vi "Initialise Panel.vi"(8 "error in":errorcluster, 9 "MHL Configuration":T6, 10 "MHL References":T5, 11 "MHL UI Data In":T2={"Status"="", "Connection Type"=enum."Ethernet", "Connected to Controller"=FALSE, "Axes Enabled"=FALSE, "Jogging Enabled"=FALSE, "X Axis MPOS"=0.0, "A Axis MPOS"=0.0, "X Axis SPEED"=0.0, "A Axis SPEED"=0.0, "Plot Laser Data"=FALSE, "MHL Status"=enum."Disconnected"} {"A Axis SPEED" format="%#_4g"; "X Axis SPEED" format="%#_4g"; "A Axis MPOS" format="%#_4g"; "X Axis MPOS" format="%#_4g"}) -> (0 "error out":errorcluster, 2 "MHL Data":T1={"MHL UI Data"={"Status"="", "Connection Type"=enum."Ethernet", "Connected to Controller"=FALSE, "Axes Enabled"=FALSE, "Jogging Enabled"=FALSE, "X Axis MPOS"=0.0, "A Axis MPOS"=0.0, "X Axis SPEED"=0.0, "A Axis SPEED"=0.0, "Plot Laser Data"=FALSE, "MHL Status"=enum."Disconnected"}, "MHL References"={"Connect to Controller Ref"=refnum, "Connection Type Ref"=refnum, "Set Parameters Ref"=refnum, "Enable Axes Ref"=refnum, "Home Axes Ref"=refnum}, "MHL Configuration"={"Fuel Control Valve Maximum"=0.0, "Fuel Control Valve Minimum"=0.0}} {"MHL UI Data"."A Axis SPEED" format="%#_4g"; "MHL UI Data"."X Axis SPEED" format="%#_4g"; "MHL UI Data"."A Axis MPOS" format="%#_4g"; "MHL UI Data"."X Axis MPOS" format="%#_4g"}, 3 "MHL UI Data Out":T2={"Status"="", "Connection Type"=enum."Ethernet", "Connected to Controller"=FALSE, "Axes Enabled"=FALSE, "Jogging Enabled"=FALSE, "X Axis MPOS"=0.0, "A Axis MPOS"=0.0, "X Axis SPEED"=0.0, "A Axis SPEED"=0.0, "Plot Laser Data"=FALSE, "MHL Status"=enum."Disconnected"} {"A Axis SPEED" format="%#_4g"; "X Axis SPEED" format="%#_4g"; "A Axis MPOS" format="%#_4g"; "X Axis MPOS" format="%#_4g"})   [LabVIEW 2020]
uses:
  controls/MHL UI Data.ctl
  TrioMotion Controller/Connection Type.ctl
  controls/MHL Status.ctl
  controls/MHL Configuration.ctl
  controls/MHL References.ctl
  controls/MHL Data.ctl
  SR-Test Med System Globals.vi
  TrioMotion Controller/TrioMotion Controller.lvlib
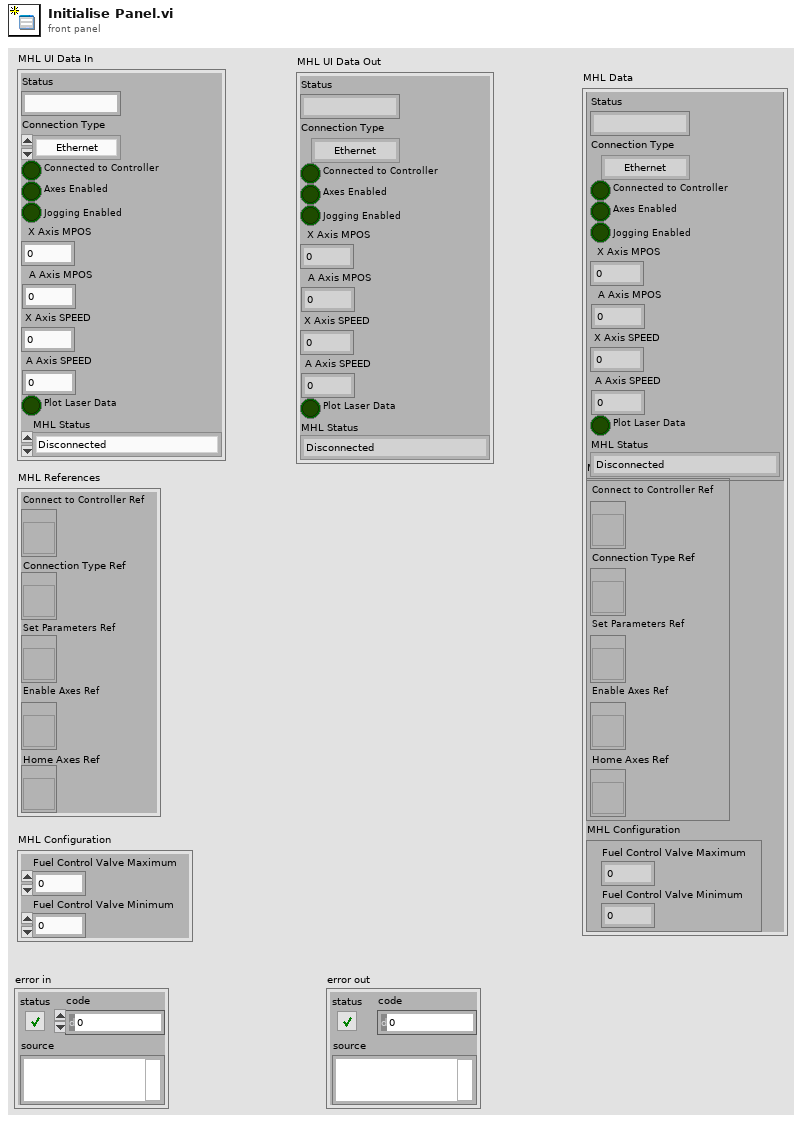
[diagram p1: front panel]
types:
  T1 = typedef "MHL Data.ctl" = cluster{"MHL UI Data":T2, "MHL References":T5, "MHL Configuration":T6}
  T2 = typedef "MHL UI Data.ctl" = cluster{"Status":string, "Connection Type":T3, "Connected to Controller":bool, "Axes Enabled":bool, "Jogging Enabled":bool, "X Axis MPOS":dbl, "A Axis MPOS":dbl, "X Axis SPEED":dbl, "A Axis SPEED":dbl, "Plot Laser Data":bool, "MHL Status":T4}
  T3 = typedef "TrioMotion Controller.lvlib/Connection Type.ctl" = enum16{"USB", "Serial", "Ethernet", "PCI", "Path", "No connection"}
  T4 = typedef "MHL Status.ctl" = enum16{"Disconnected", "Connecting", "Connected", "Axes Enabled", "Machine Running", "Shutdown"}
  T5 = typedef "MHL References.ctl" = cluster{"Connect to Controller Ref":refnum<vi>, "Connection Type Ref":refnum<vi>, "Set Parameters Ref":refnum<vi>, "Enable Axes Ref":refnum<vi>, "Home Axes Ref":refnum<vi>}
  T6 = typedef "MHL Configuration.ctl" = cluster{"Fuel Control Valve Maximum":dbl, "Fuel Control Valve Minimum":dbl}
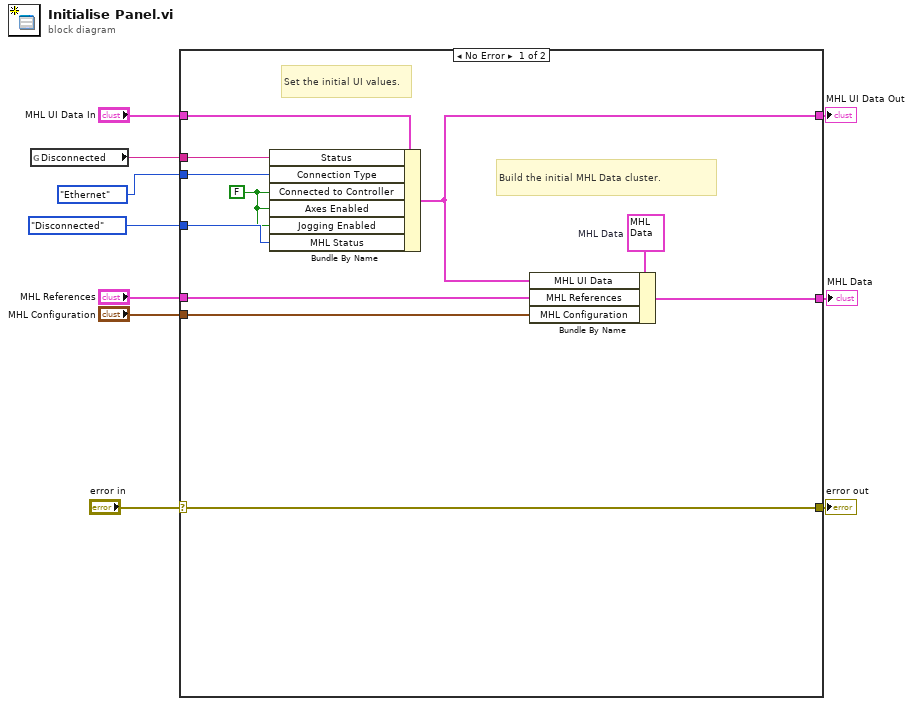
[diagram p0: block diagram]
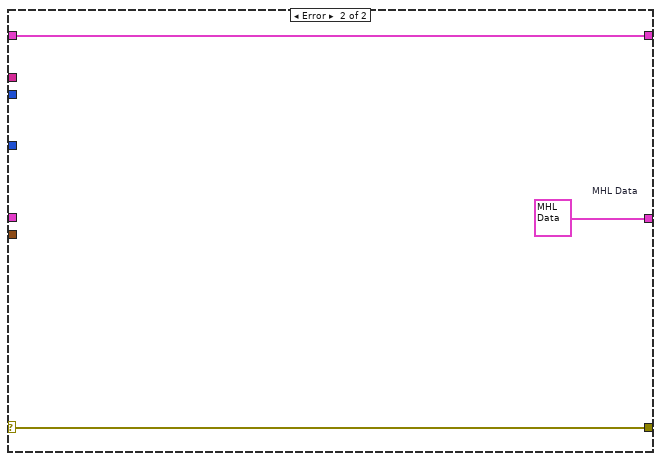
[diagram p2: hidden frame]
diagram:
  n1 = global read "SR-Test Med System Globals.vi" "Disconnected"() -> (w4:string)
  n2 = case shown="No Error" "error in" {
    selector: "error in" -> [w15 w24]
    tunnel: [w15 w24] -> w9
    tunnel: [w17 w23] -> w7
    tunnel: "MHL UI Data In" -> [w21 w23]
    tunnel: [w18 w22] -> w6
    tunnel: MHL_Status."Disconnected" ("MHL Status") -> [w13 _]
    tunnel: w4 -> [w20 _]
    tunnel: "MHL References" -> [w14 _]
    tunnel: "MHL Configuration" -> [w16 _]
    tunnel: Connection_Type."Ethernet" ("Value") -> [w11 _]
    frame No Error {
      w12 = FALSE ("Axes Enabled")
      w19 = T1 {"MHL UI Data"={"Status"="", "Connection Type"=enum."Ethernet", "Connected to Controller"=FALSE, "Axes Enabled"=FALSE, "Jogging Enabled"=FALSE, "X Axis MPOS"=0.0, "A Axis MPOS"=0.0, "X Axis SPEED"=0.0, "A Axis SPEED"=0.0, "Plot Laser Data"=FALSE, "MHL Status"=enum."Disconnected"}, "MHL References"={"Connect to Controller Ref"=refnum, "Connection Type Ref"=refnum, "Set Parameters Ref"=refnum, "Enable Axes Ref"=refnum, "Home Axes Ref"=refnum}, "MHL Configuration"={"Fuel Control Valve Maximum"=0.0, "Fuel Control Valve Minimum"=0.0}}  # MHL Data
      # "Build the initial MHL Data cluster."
      # "Set the initial UI values."
      n3 = Bundle By Name(cluster=w21, "Status"=w20, "Connection Type"=w11, "Connected to Controller"=w12, "Axes Enabled"=w12, "Jogging Enabled"=w12, "MHL Status"=w13) -> (w17:T2)
      n4 = Bundle By Name(cluster=w19, "MHL UI Data"=w17, "MHL References"=w14, "MHL Configuration"=w16) -> (w18:T1)
    }
    frame Error {
      w22 = T1 {"MHL UI Data"={"Status"="", "Connection Type"=enum."Ethernet", "Connected to Controller"=FALSE, "Axes Enabled"=FALSE, "Jogging Enabled"=FALSE, "X Axis MPOS"=0.0, "A Axis MPOS"=0.0, "X Axis SPEED"=0.0, "A Axis SPEED"=0.0, "Plot Laser Data"=FALSE, "MHL Status"=enum."Disconnected"}, "MHL References"={"Connect to Controller Ref"=refnum, "Connection Type Ref"=refnum, "Set Parameters Ref"=refnum, "Enable Axes Ref"=refnum, "Home Axes Ref"=refnum}, "MHL Configuration"={"Fuel Control Valve Maximum"=0.0, "Fuel Control Valve Minimum"=0.0}}  # MHL Data
    }
  }
  "error out" <- w9
  "MHL UI Data Out" <- w7
  "MHL Data" <- w6
